vi "PH_Sound.ProcEvents.vi"(0 "i ref in":refnum<vi>, 5 "error in (no error)":errorcluster) -> (14 "i ref out":refnum<vi>, 19 "error out":errorcluster)   [LabVIEW 2014, in "PH_Sound.lvlib"]
doc: "This method is used to define the events the object will listen to. Add your own events here."
uses:
  PH_Sound.lvlib
  CSCore/BaseProcess/BaseProcess.event definition.ctl
  CSCore/CAEObj/CAEObj.event definition.ctl
  CSCore/BaseProcess/BaseProcess.descriptor string definition.ctl
  CSCore/BaseProcess/BaseProcess.lvlib
  CSCore/CAEObj/CAEObj.lvlib
  PH_Common/PH_Common.lvlib
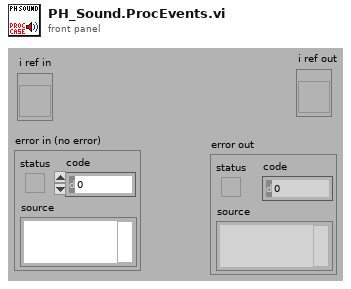
[diagram p1: front panel]
types:
  T1 = typedef "BaseProcess.lvlib/BaseProcess.event definition.ctl" = cluster{"CAEEvtDef":T2, "Data Descriptor":T3}
  T2 = typedef "CAEObj.lvlib/CAEObj.event definition.ctl" = cluster{"URL":string, "enable":bool, "ignoreResID":bool}
  T3 = typedef "BaseProcess.lvlib/BaseProcess.descriptor string definition.ctl" = string
  T4 = typedef "PH_Common.lvlib/PH_DIM.Event Declarer.ctl" = cluster{"Service Name":string, "Selector":string}
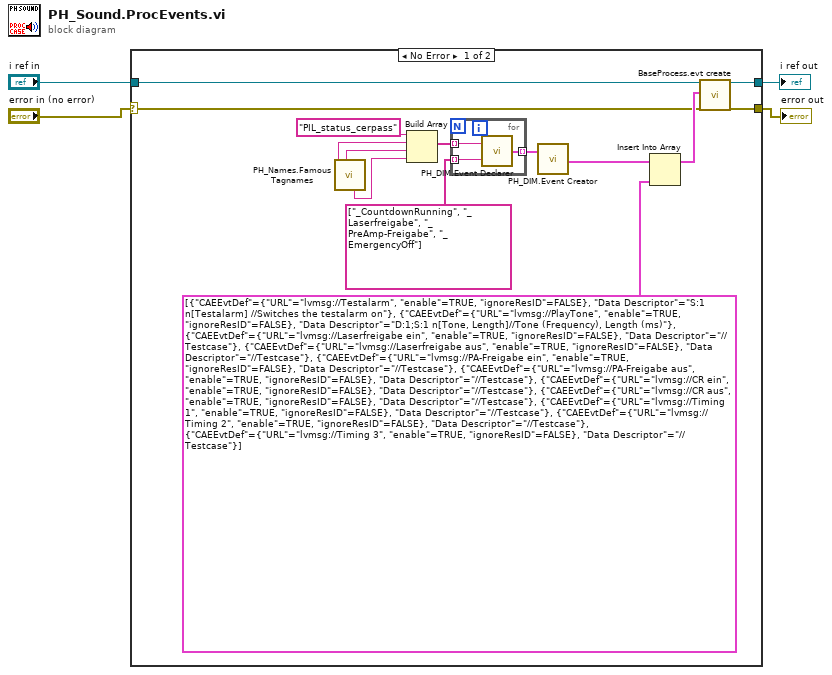
[diagram p0: block diagram]
diagram:
  n1 = case shown="No Error" "error in (no error)" {
    selector: "error in (no error)" -> [w8 w22]
    tunnel: "i ref in" -> [w9 w23]
    tunnel: [w17 w23] -> w3
    tunnel: [w16 w22] -> w2
    frame No Error {
      n2 = call "PH_Names.Famous Tagnames.vi"() -> ("Laser Enabling.DIM Service Name"=w6:string, "PreAmp Enabling.DIM Service Name"=w5:string, "Emergency Off.DIM Service Name"=w7:string)  [unwired: 2 in, 6 out]
      n3 = Build Array("PIL_status_cerpass" ("DIM Service Name Status CerPass"), w6, w5, w7) -> (w15:string[])
      n4 = for {
        tunnel: w15 -> [w21] mode=indexing
        tunnel: [w20] -> w14 mode=indexing
        tunnel: string[] ["_CountdownRunning", "_Laserfreigabe", "_PreAmp-Freigabe", "_EmergencyOff"] -> [w19] mode=indexing
        n5 = call "PH_DIM.Event Declarer.vi"("Selector"=w19, "Service Name"=w21) -> ("declared DIM Event"=w20:T4)
      }
      n6 = call "PH_DIM.Event Creator.vi"("Trendmessage Services"=w14) -> ("DIM Service Events"=w13:T1[])  [unwired: 18 in]
      n7 = Insert Into Array(array=w13, new element=T1[] [{"CAEEvtDef"={"URL"="lvmsg://Testalarm", "enable"=TRUE, "ignoreResID"=FALSE}, "Data Descriptor"="S:1 n[Testalarm] //Switches the testalarm on"}, {"CAEEvtDef"={"URL"="lvmsg://PlayTone", "enable"=TRUE, "ignoreResID"=FALSE}, "Data Descriptor"="D:1;S:1 n[Tone, Length]//Tone (Frequency), Length (ms)"}, {"CAEEvtDef"={"URL"="lvmsg://Laserfreigabe ein", "enable"=TRUE, "ignoreResID"=FALSE}, "Data Descriptor"="//Testcase"}, {"CAEEvtDef"={"URL"="lvmsg://Laserfreigabe aus", "enable"=TRUE, "ignoreResID"=FALSE}, "Data Descriptor"="//Testcase"}, {"CAEEvtDef"={"URL"="lvmsg://PA-Freigabe ein", "enable"=TRUE, "ignoreResID"=FALSE}, "Data Descriptor"="//Testcase"}, {"CAEEvtDef"={"URL"="lvmsg://PA-Freigabe aus", "enable"=TRUE, "ignoreResID"=FALSE}, "Data Descriptor"="//Testcase"}, {"CAEEvtDef"={"URL"="lvmsg://CR ein", "enable"=TRUE, "ignoreResID"=FALSE}, "Data Descriptor"="//Testcase"}, {"CAEEvtDef"={"URL"="lvmsg://CR aus", "enable"=TRUE, "ignoreResID"=FALSE}, "Data Descriptor"="//Testcase"}, {"CAEEvtDef"={"URL"="lvmsg://Timing 1", "enable"=TRUE, "ignoreResID"=FALSE}, "Data Descriptor"="//Testcase"}, {"CAEEvtDef"={"URL"="lvmsg://Timing 2", "enable"=TRUE, "ignoreResID"=FALSE}, "Data Descriptor"="//Testcase"}, {"CAEEvtDef"={"URL"="lvmsg://Timing 3", "enable"=TRUE, "ignoreResID"=FALSE}, "Data Descriptor"="//Testcase"}] ("new events")) -> (w18:T1[])  [unwired: 1 in]
      n8 = call "BaseProcess.evt create.vi"("i ref in"=w9, "newEvents"=w18, "error in (no error)"=w8) -> ("i ref out"=w17:refnum<vi>, "error out"=w16:errorcluster)  [unwired: 13 in, 2 out]
    }
    frame Error {
    }
  }
  "i ref out" <- w3
  "error out" <- w2
